vi "ToJason.vi"(8 "error in (no error)":errorcluster, 11 "Flags in":refnum<class "Flags.lvclass">) -> (0 "error out":errorcluster, 3 "Flags out":refnum<class "Flags.lvclass">)   [LabVIEW 2015, in "Flags.lvclass"]
uses:
  Flags.lvclass
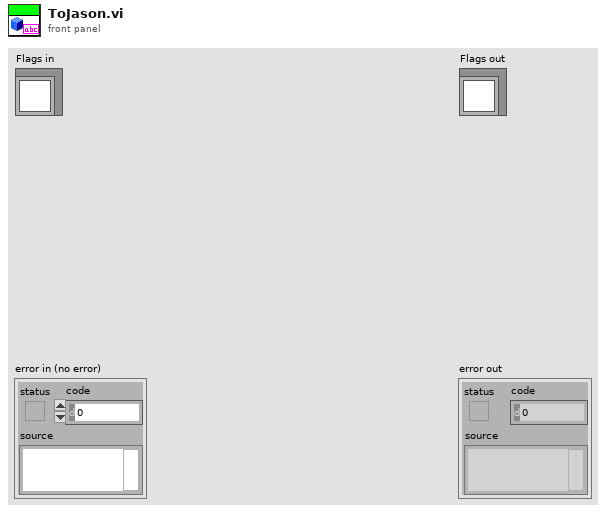
[diagram p1: front panel]
types:
  T1 = typedef "Flags.lvclass/ColorEnum.ctl" = enum8{"Red", "Blue", "Green", "Yellow"}
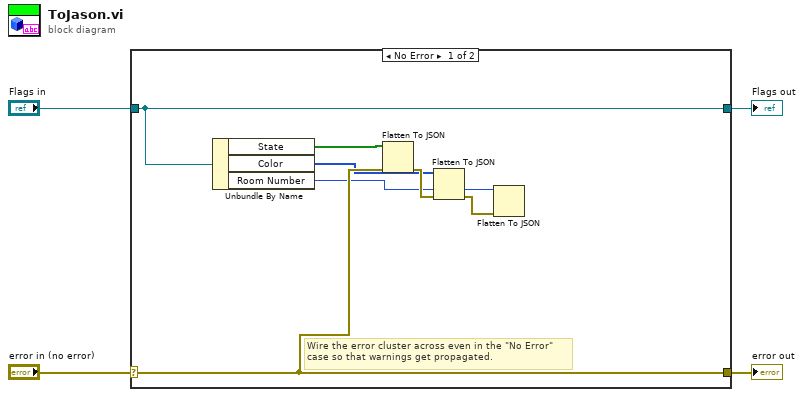
[diagram p0: block diagram]
diagram:
  n1 = case shown="No Error" "error in (no error)" {
    selector: "error in (no error)" -> [w9 w13]
    tunnel: [w9 w13] -> w3
    tunnel: [w11 w12] -> w1
    tunnel: "Flags in" -> [w11 w12]
    frame No Error {
      # "Wire the error cluster across even in the \"No Error\"\ncase so that warnings get propagated."
      n2 = Unbundle By Name(w11) -> ("State"=w10:bool[], "Color"=w6:T1[], "Room Number"=w5:u32)
      n3 = Flatten To JSON(anything=w10, error in (no error)=w9) -> (11:w8:errorcluster)  [unwired: 1 in, 1 out]
      n4 = Flatten To JSON(anything=w6, error in (no error)=w8) -> (11:w7:errorcluster)  [unwired: 1 in, 1 out]
      n5 = Flatten To JSON(anything=w5, error in (no error)=w7) -> ()  [unwired: 1 in, 2 out]
    }
    frame Error {
    }
  }
  "error out" <- w3
  "Flags out" <- w1
